vi "VarGlobal.vi"() -> ()   [LabVIEW 2018]
panel:
  out "HumidityGraph":dbl[](array[numeric])
  out "PressureGraph":dbl[](array[numeric])
  out "TemperatureGraph":dbl[](array[numeric])
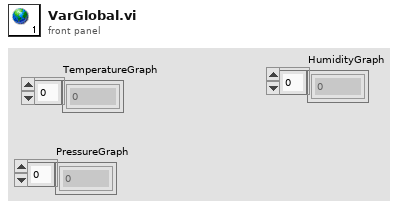
[diagram p1: front panel]
diagram:
